vi "TCP_server.vi"(7 "Flow Control":enum16{"Listen", "Read", "Write", "Close"}(ring), 8 "error in":errorcluster, 9 "Send Message":string, 10 "Local Server Port":u16, 11 "service name":string) -> (0 "error out":errorcluster, 1 "Message":string)   [LabVIEW 2012]
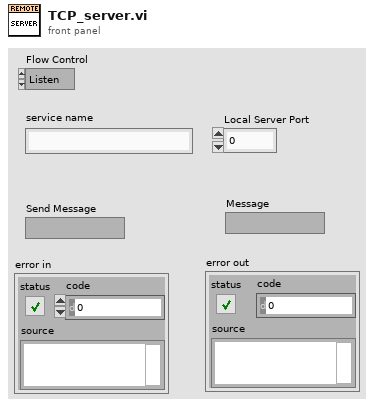
[diagram p1: front panel]
types:
  T1 = enum16{"Standard", "Buffered", "CRLF", "Immediate"}
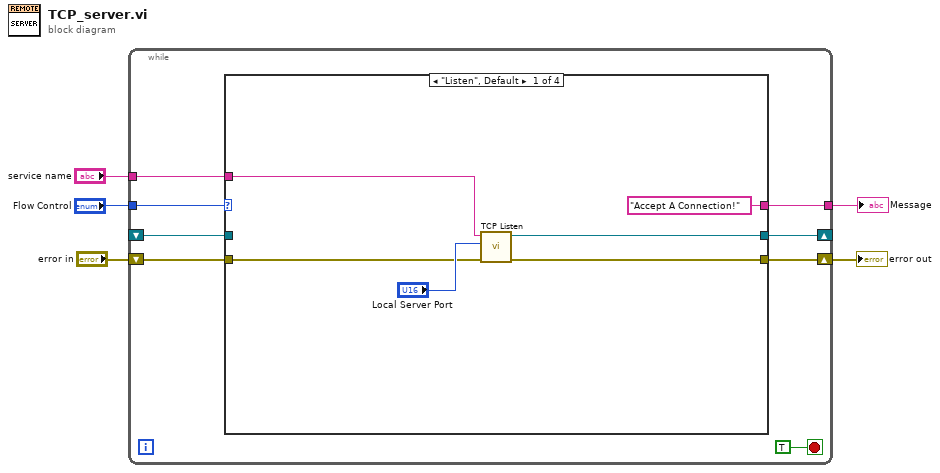
[diagram p0: block diagram]
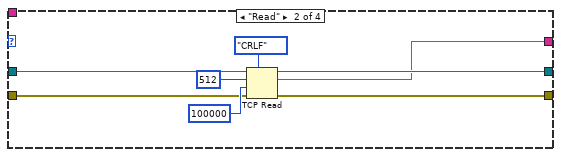
[diagram p2: hidden frame]
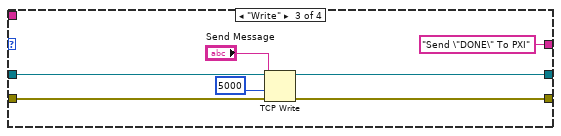
[diagram p3: hidden frame]
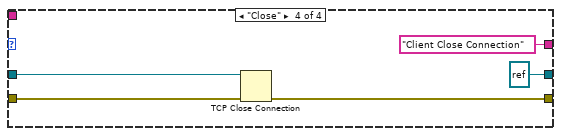
[diagram p4: hidden frame]
diagram:
  n1 = while {
    shift-right: [w11] -> w4
    shift-left: "error in" -> [w12]
    shift-right: [w10] -> _
    shift-left: _ -> [w9]
    tunnel: "Flow Control" -> [w8]
    tunnel: "service name" -> [w7]
    tunnel: [w6] -> w1
    stop <- TRUE stop-if-true
    n2 = case shown="\"Listen\", Default" w8 {
      tunnel: w12 -> [w18 w21 w30 w38]
      tunnel: [w17 w22 w29 w37] -> w11
      tunnel: [w16 w23 w31 refnum<k5> refnum ("connection ID")] -> w10
      tunnel: w9 -> [_ w24 w32 w39]
      tunnel: w7 -> [w15 _ _ _]
      tunnel: ["Accept A Connection!" ("data out") w20 "Send \"DONE\" To PXI" ("data out") "Client Close Connection" ("data out")] -> w6
      frame "Listen", Default {
        n3 = call <vilib>:"TCP Listen.vi"("error in (no error)"=w18, "port"="Local Server Port", "service name"=w15) -> ("error out"=w17:errorcluster, "connection ID"=w16:refnum<k5>)  [unwired: 4 in, 3 out]
      }
      frame "Read" {
        n4 = TCP Read(connection ID=w24, bytes to read=512, error in (no error)=w21, 7:T1."CRLF" ("mode (standard)"), 9:100000 ("timeout ms (25000)")) -> (connection ID out=w23:refnum<k5>, data out=w20:string, error out=w22:errorcluster)
      }
      frame "Write" {
        n5 = TCP Write(connection ID=w32, data in="Send Message", error in (no error)=w30, 9:5000 ("timeout ms (25000)")) -> (connection ID out=w31:refnum<k5>, error out=w29:errorcluster)  [unwired: 1 out]
      }
      frame "Close" {
        n6 = TCP Close Connection(connection ID=w39, error in (no error)=w38) -> (error out=w37:errorcluster)  [unwired: 1 in, 1 out]
      }
    }
  }
  "error out" <- w4
  "Message" <- w1
